vi "MVE Alias Browse.vi"(10 "Item Path":string, 11 "InitPath":string) -> (3 "outPath":string)   [LabVIEW 2016]
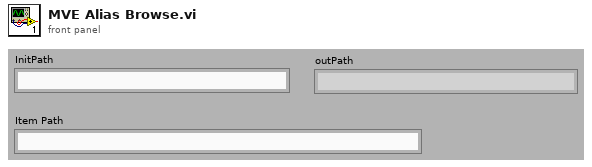
[diagram p1: front panel]
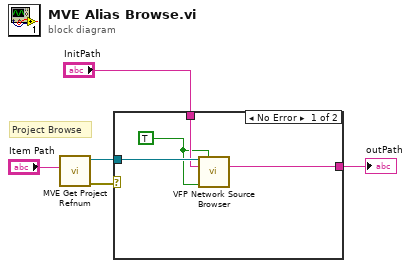
[diagram p0: block diagram]
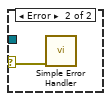
[diagram p2: hidden frame]
diagram:
  # "Project Browse"
  n1 = call <resource>:"MVE Get Project Refnum.vi"("Full Path"="Item Path") -> ("error out"=w2:errorcluster, "Project Refnum"=w3:refnum<vi>)  [unwired: 2 in, 7 out]
  n2 = case shown="No Error" w2 {
    selector: w2 -> [_ w10]
    tunnel: [w9 _] -> w5
    tunnel: w3 -> [w8 _]
    tunnel: "InitPath" -> [w7 _]
    frame No Error {
      w6 = TRUE ("IO Vars only?")
      n3 = call <resource>:"VFP Network Source Browser.vi"("Project Refnum"=w8, "Include IO Vars? (F)"=w6, "InitPath"=w7, "Include IO Aliases? (F)"=w6) -> ("outPath"=w9:string)  [unwired: 3 in, 8 out]
    }
    frame Error {
      n4 = call <vilib>:"Simple Error Handler.vi"("error in (no error)"=w10) -> ()  [unwired: 1 in, 8 out]
    }
  }
  "outPath" <- w5
